vi "Read Bit.vi"(7 "Specified Num in":u8=1, 8 "error in (no error)":errorcluster caption="error in", 10 "Address":u16=65535 format="%.0x", 11 "Port Selection Info In":T1={"Port Name"="", "Amplifier Num"=1, "Baud Rate"=38400, "Char Formation"=enum."0"} {"Baud Rate" items=["38400"=38400, "19200"=19200, "9600"=9600, "115200"=0]; "Amplifier Num" max=31}) -> (0 "error out":errorcluster, 2 "bits array":bool[](array[boolean]), 3 "Port Selection Info Out":T1={"Port Name"="", "Amplifier Num"=1, "Baud Rate"=38400, "Char Formation"=enum."0"} {"Baud Rate" items=["38400"=38400, "19200"=19200, "9600"=9600, "115200"=0]; "Amplifier Num" max=31})   [LabVIEW 2014, in "ALPHA5 RS485.lvlib"]
uses:
  ALPHA5 RS485.lvlib
  typedefs/Port Selection Info.ctl
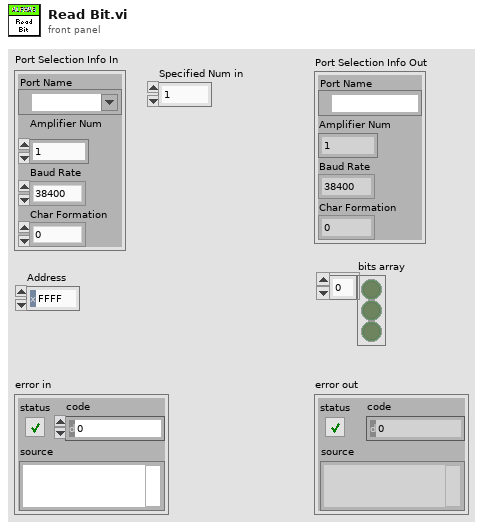
[diagram p1: front panel]
types:
  T1 = typedef "ALPHA5 RS485.lvlib/Port Selection Info.ctl" = cluster{"Port Name":refnum<visa-resource-name>, "Amplifier Num":u8, "Baud Rate":u32, "Char Formation":enum16{"0", "1", "2", "3", "4", "5"}}
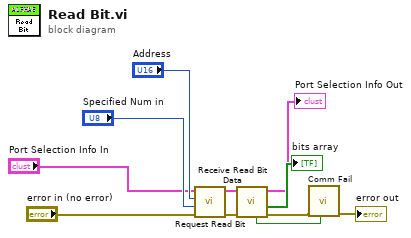
[diagram p0: block diagram]
diagram:
  n1 = call "Request Read Bit.vi"("error in (no error)"="error in (no error)", "Specified Num in"="Specified Num in", "Address"="Address", "Port Selection Info"="Port Selection Info In") -> ("error out"=w10:errorcluster, "Port Selection Info Out"=w11:T1)  [unwired: 5 in, 1 out]
  n2 = call "Receive Read Bit Data.vi"("error in (no error)"=w10, "Port Selection Info"=w11) -> ("error out"=w4:errorcluster, "bits array"=→"bits array":bool[], "Port Selection Info Out"=→"Port Selection Info Out":T1, "CRC Match"=w2:bool)  [unwired: 3 in, 3 out]
  n3 = call "Comm Fail.vi"("CRC Match"=w2, "error in (no error)"=w4) -> ("error out"=→"error out":errorcluster)  [unwired: 9 in]
